vi "Basic Time Conversion.vi"(6 "Units":string(combo), 11 "Time IN":dbl) -> (3 "Time OUT (s)":dbl)   [LabVIEW 2021]
doc: "This converts human accuracy time units to seconds.\n\n60 seconds in a minute\n60 minutes in an hour\n24 hours in a day\n365 days in a year"
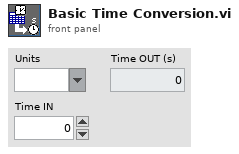
[diagram p1: front panel]
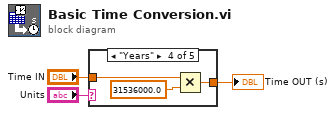
[diagram p0: block diagram]
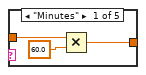
[diagram p2: hidden frame]
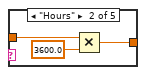
[diagram p3: hidden frame]
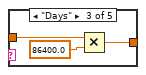
[diagram p4: hidden frame]
diagram:
  n1 = case shown="\"Years\"" "Units" {
    tunnel: "Time IN" -> [w5 w9 w12 w15 w16]
    tunnel: [w4 w8 w10 w13 w16] -> w1
    frame "Minutes" {
      n2 = Multiply(x=w5, y=60.0) -> (x*y=w4:dbl)
    }
    frame "Hours" {
      n3 = Multiply(x=w9, y=3600.0) -> (x*y=w8:dbl)
    }
    frame "Days" {
      n4 = Multiply(x=w12, y=86400.0) -> (x*y=w10:dbl)
    }
    frame "Years" {
      n5 = Multiply(x=w15, y=31536000.0) -> (x*y=w13:dbl)
    }
    frame Default {
    }
  }
  "Time OUT (s)" <- w1
